vi "convert type defs to channels.vi"(11 "fixed channel configuration":refnum<class "control module configuration.lvclass">) -> (0 "error out":errorcluster, 3 "Array out":refnum<class "TBM channel.lvclass">[](array[class]))   [LabVIEW 2013, in "control module configuration.lvclass"]
uses:
  control module configuration.lvclass
  <vilib>/NI/Tag Bus Module Framework/channel/TBM channel.lvclass
  <vilib>/regexp/Match Regular Expression.xnode
  <vilib>/NI/Configuration Framework/NISE_CEF_TreeControl.lvlib
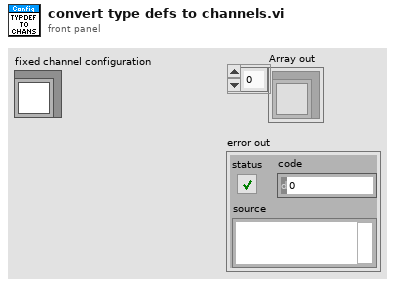
[diagram p1: front panel]
types:
  T1 = typedef "TBM channel.lvclass/channel classification.ctl" = enum16{"input data", "output data", "processing parameter", "processing result"}
  T2 = typedef "tag bus.lvlib/tag descriptor.lvclass/Data Type.ctl" = enum16{"Double", "Single", "I64", "I32", "I16", "I8", "U64", "U32", "U16", "U8", "Boolean", "String", "Array of Double", "Array of Single", "Array of I64", "Array of I32", "Array of I16", "Array of I8", "Array of U64", "Array of U32", "Array of U16", "Array of U8", "Array of Boolean", "Array of String"}
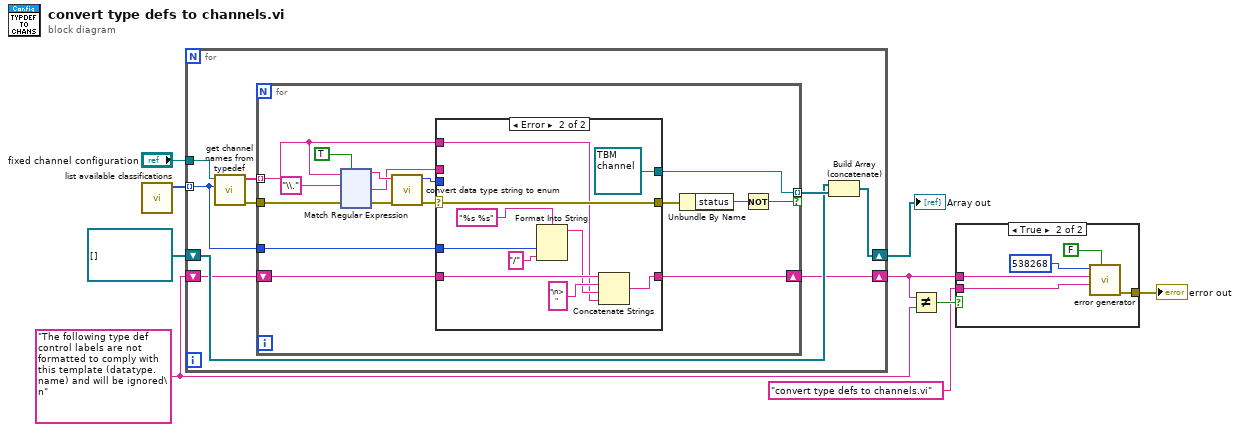
[diagram p0: block diagram]
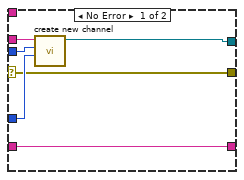
[diagram p3: hidden frame]
diagram:
  w6 = "The following type def control labels are not formatted to comply with this template (datatype.name) and will be ignored\n"
  n1 = call <vilib>:"list available classifications.vi"() -> ("supported types"=w1:T1[])  [unwired: 11 in]
  n2 = for {
    shift-right: [w17] -> w5
    shift-left: refnum<class "TBM channel.lvclass">[] [] -> [w16]
    shift-right: [w14] -> w8
    shift-left: w6 -> [w15]
    tunnel: "fixed channel configuration" -> [w12]
    tunnel: w1 -> [w11] mode=indexing
    n3 = call "get channel names from typedef.vi"("channel classification"=w11, "fixed channel configuration"=w12) -> ("error out"=w13:errorcluster, "Channel Names"=w10:string[])  [unwired: 8 in]
    n4 = for {
      tunnel: w11 -> [w33]
      tunnel: [w34] -> w18 mode=indexing if=w24
      tunnel: w10 -> [w21] mode=indexing
      shift-right: [w19] -> w14
      shift-left: w15 -> [w20]
      tunnel: w13 -> [w30]
      n5 = xnode "Match Regular Expression"("input string"=w21, "regular expression"="\\.", "error in"=w30, "ignore case? (F)"=TRUE) -> ("before match"=w28:string, "after match"=w27:string, "error out"=w29:errorcluster)  [unwired: 2 in, 2 out]
      n6 = call "convert data type string to enum.vi"("error in"=w29, "Data Type String"=w28) -> ("error out"=w26:errorcluster, "Data Type Enum"=w22:T2)  [unwired: 8 in]
      n7 = case shown="Error" w26 {
        selector: w26 -> [w152 w163]
        tunnel: w33 -> [w154 w159]
        tunnel: [w152 w163] -> w25
        tunnel: [w153 refnum<class "TBM channel.lvclass"> refnum ("channel")] -> w34
        tunnel: w27 -> [w151 _]
        tunnel: w22 -> [w150 _]
        tunnel: w21 -> [_ w155]
        tunnel: w20 -> [w149 w162]
        tunnel: [w149 w161] -> w19
        frame No Error {
          n8 = call <vilib>:"create new channel.vi"("channel classification"=w154, "data type"=w150, "channel name"=w151) -> ("channel"=w153:refnum<class "TBM channel.lvclass">)  [unwired: 8 in]
        }
        frame Error {
          n9 = Format Into String(format string="%s %s", w159, "/") -> (resulting string=w156:string)  [unwired: 2 in, 1 out]
          n10 = Concatenate Strings(w162, "\n> " ("string"), w156, w155) -> (w161:string)
        }
      }
      n11 = Unbundle By Name(w25) -> ("status"=w23:bool)
      n12 = Not(x=w23) -> (.not. x?=w24:bool)
    }
    n13 = Build Array (concatenate)(w16, w18) -> (w17:refnum<class "TBM channel.lvclass">[])
  }
  "Array out" <- w5
  n14 = Not Equal?(x=w8, y=w6) -> (x != y?=w7:bool)
  n15 = case shown="True" w7 {
    tunnel: w8 -> [_ w168]
    tunnel: [_ w169] -> w9
    tunnel: "convert type defs to channels.vi" ("source") -> [_ w165]
    frame False {
    }
    frame True {
      n16 = call <vilib>:"error generator.vi"("error (T)"=FALSE, "source"=w165, "append error message"=w168, "error code (0)"=538268) -> ("error out"=w169:errorcluster)  [unwired: 5 in]
    }
  }
  "error out" <- w9
